vi "Write Deadband.vi"(8 "error in (no error)":errorcluster, 10 "Deadband":cluster{"LO":dbl, "HI":dbl}, 11 "Level Controller in":refnum<class "Level Controller.lvclass">) -> (0 "error out":errorcluster, 3 "Level Controller out":refnum<class "Level Controller.lvclass">)   [LabVIEW 2012, in "Level Controller.lvlib" / "Level Controller.lvclass"]
uses:
  Level Controller.lvclass
  Level Controller.lvclass/Level Controller.ctl
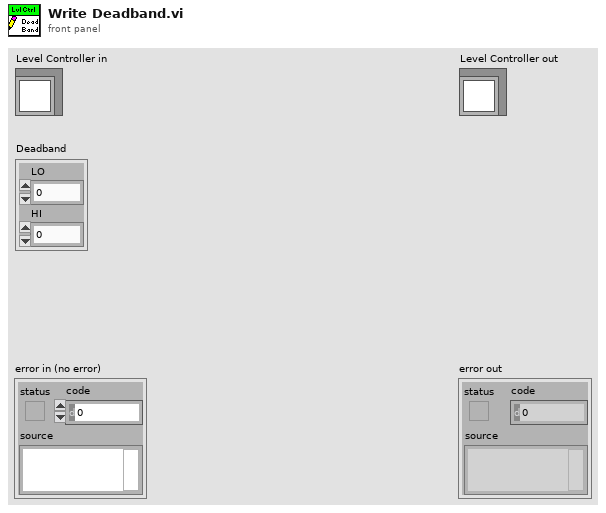
[diagram p1: front panel]
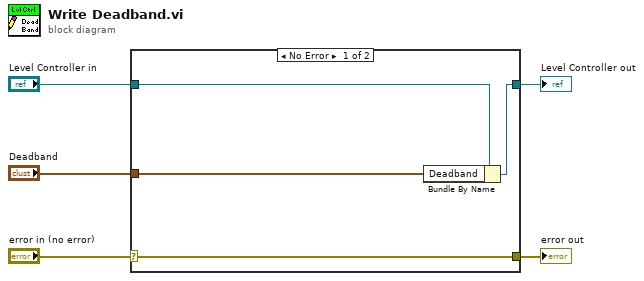
[diagram p0: block diagram]
diagram:
  n1 = case shown="No Error" "error in (no error)" {
    selector: "error in (no error)" -> [w9 w10]
    tunnel: [w9 w10] -> w4
    tunnel: [w7 w11] -> w2
    tunnel: "Level Controller in" -> [w8 w11]
    tunnel: "Deadband" -> [w6 _]
    frame No Error {
      n2 = Bundle By Name(cluster=w8, "Deadband"=w6) -> (w7:refnum<class "Level Controller.lvclass">)
    }
    frame Error {
    }
  }
  "error out" <- w4
  "Level Controller out" <- w2
